vi "11 - Design Pattern - When Generation Rate exceeds Handling Rate (Accumulator).vi"() -> ()   [LabVIEW 2012]
uses:
  <vilib>/Utility/miscctls.llb/LVPoint32TypeDef.ctl
  <vilib>/Utility/miscctls.llb/LVPointTypeDef.ctl
  <vilib>/event_ctls.llb/lveventtype.ctl
panel:
  out "Canvas":picture
  in  "Erase":bool
  out "Events Handled per Update":dbl format="%.02f"
  in  "Handler Throttle Period":u32(ring)=50 items=["None"=0, "50msec"=50, "200msec"=200, "500msec"=500]
  out "Processor Usage":sgl(graph)
  out "Initial Coords":T1
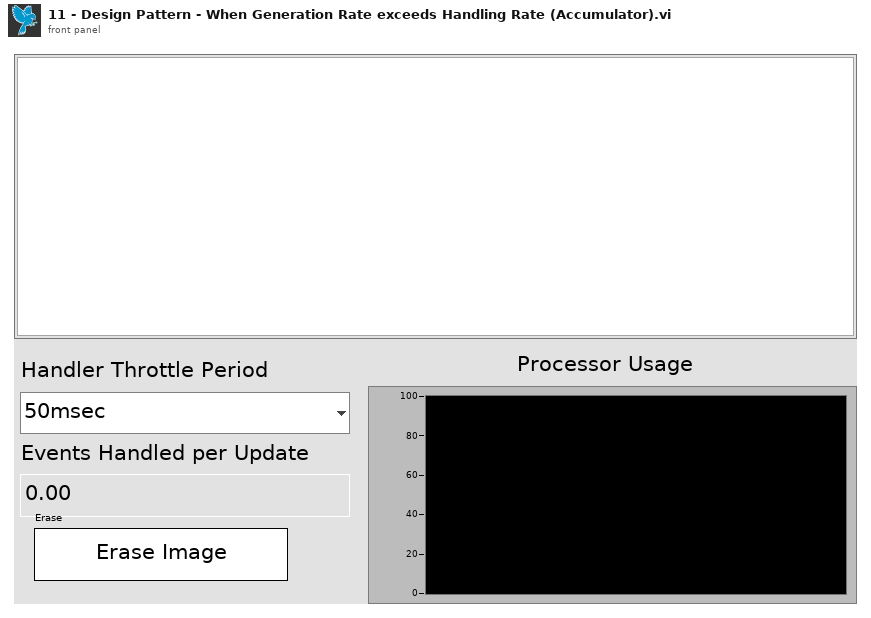
[diagram p1: front panel]
types:
  T1 = typedef "LVPoint32TypeDef.ctl" = cluster{"Horizontal":i32, "Vertical":i32}
  T2 = typedef "LVPointTypeDef.ctl" = cluster{"Horizontal":i16, "Vertical":i16}
  T3 = enum16{"Currently Painting", "Currently Zooming", "No Action"}
  T4 = typedef "lveventtype.ctl" = enum32{"Null", "Timeout", "Annotation Menu Selection", "Annotation Menu Selection?", "App Instance Close", "App Instance Close?", "Autoscale Range Change", "Cell Edit", "Cell Edit?", "Cursor Grab", "Cursor Grab?", "Cursor Menu Selection", "Cursor Menu Selection?", "Cursor Move", "Cursor Release", "Data Change", "Direction Change", "Display State Change", "Drag Ended", "Drag Enter", "Drag Leave", "Drag Over", "Drag Source Update", "Drag Starting", "Drag Starting?", "Drop", "Exec State Change", "Key Down", "Key Down?", "Key Repeat", "Key Repeat?", "Key Up", "Listbox Double Click", "Menu Activation?", "Menu Selection (App)", "Menu Selection? (App)", "Menu Selection (User)", "Mouse Down", "Mouse Down?", "Mouse Enter", "Mouse Leave", "Mouse Move", "Mouse Up", "NI Security User Change (App)", "Pane Size", "Panel Close", "Panel Close?", "Panel Resize", "Plot Attribute Change", "Scale Range Change", "Shortcut Menu Activation?", "Shortcut Menu Selection (App)", "Shortcut Menu Selection? (App)", "Shortcut Menu Selection (User)", "Tree Double Click", "Tree Drag", "Tree Drag?", "Tree Drop", "Tree Drop?", "Tree Item Close", "Tree Item Close?", "Tree Item Open", "Tree Item Open?", "Value Change"}
  T5 = cluster{"Width":u16, "Style":enum32{"Solid", "Dash", "Dot", "DashDot", "DashDotDot"}}
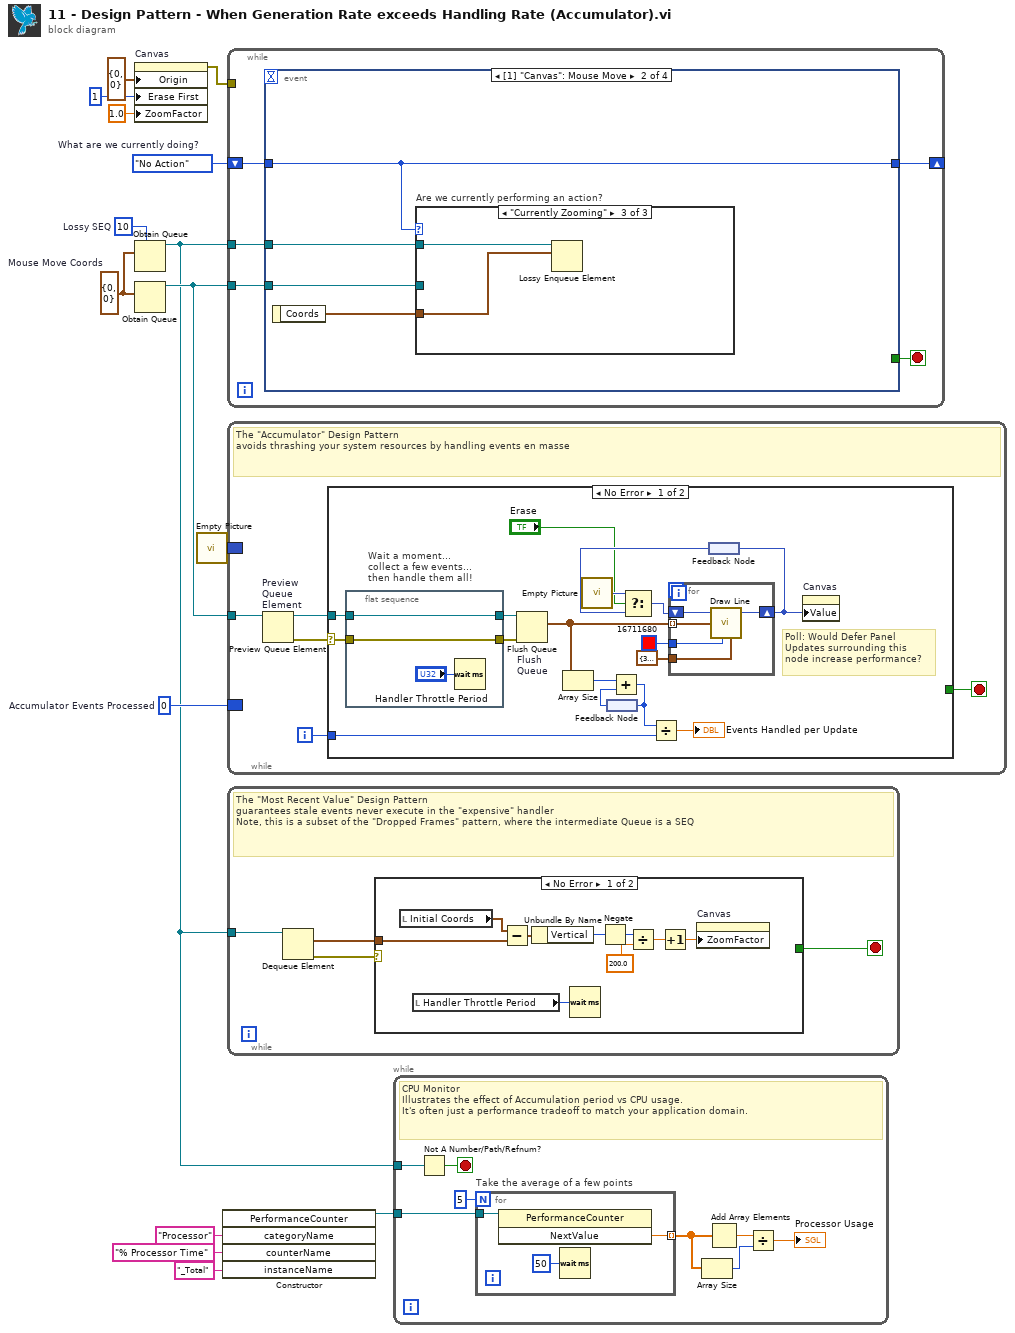
[diagram p0: block diagram]
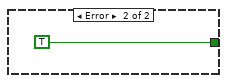
[diagram p2: hidden frame]
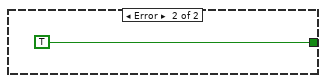
[diagram p3: hidden frame]
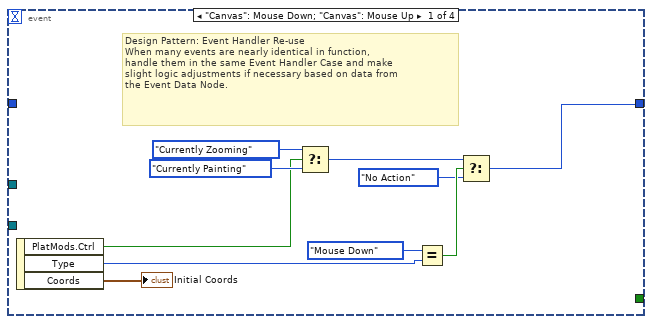
[diagram p4: hidden frame]
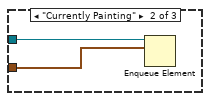
[diagram p6: hidden frame]
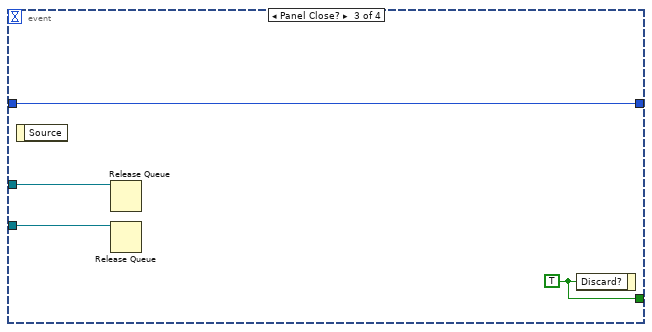
[diagram p7: hidden frame]
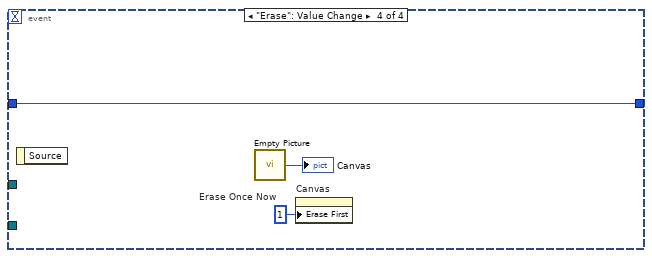
[diagram p8: hidden frame]
diagram:
  w6 = 0  # Accumulator Events Processed
  w14 = 10  # Lossy SEQ
  w15 = T3."No Action"  # What are we currently doing?
  w13 = T1 {"Horizontal"=0, "Vertical"=0}  # Mouse Move Coords
  n1 = property on="Canvas" class="Pict"("Origin"=T2 {"Horizontal"=0, "Vertical"=0}, "Erase First"=u8 1, "ZoomFactor"=sgl 1.0 ("Zoom Factor")) -> (error out=w11:errorcluster)  [unwired: 2 in, 1 out]
  n2 = Obtain Queue(max queue size (-1, unlimited)=w14, element data type=w13) -> (queue out=w2:refnum<queue>)  [unwired: 3 in, 2 out]
  n3 = Obtain Queue(element data type=w13) -> (queue out=w9:refnum<queue>)  [unwired: 4 in, 2 out]
  n4 = call "Empty Picture"() -> ("empty picture"=w10:picture)
  n5 = constructor class="PerformanceCounter"("categoryName"="Processor", "counterName"="% Processor Time", "instanceName"="_Total") -> (reference out=w3:refnum<k24>)  [unwired: 3 in, 5 out]
  n6 = while {
    shift-right: [w19] -> _
    shift-left: w15 -> [w20]
    tunnel: w9 -> [w17]
    tunnel: w2 -> [w16]
    tunnel: w11 -> [_]
    stop <- w18 stop-if-true
    n7 = event shown="[1] \"Canvas\": Mouse Move" {
      selector: _ -> [_ _ _ _]
      dyn-events: _ -> [_ _ _ _]
      timeout: _ -> [_ _ _ _]
      tunnel: w20 -> [_ w32 w41 w45]
      tunnel: [w27 w32 w41 w45] -> w19
      tunnel: [_ _ w42 _] -> w18
      tunnel: w17 -> [_ w34 w39 _]
      tunnel: w16 -> [_ w31 w40 _]
      event "Canvas": Mouse Down; "Canvas": Mouse Up {
        # "Design Pattern: Event Handler Re-use\nWhen many events are nearly identical in function,\nhandle them in the same Event Handler Case and make\nslight logic adjustments if necessary based on data from\nthe Event Data Node."
        n8 = event-data() -> ("PlatMods.Ctrl"=w21:bool, "Type"=w29:T4, "Coords"=→"Initial Coords":T1)  [unwired: 1 in]
        n9 = Select(t=T3."Currently Zooming", s=w21, f=T3."Currently Painting") -> (s? t:f=w25:T3)
        n10 = Equal?(x=lveventtype."Mouse Down" ("Type"), y=w29) -> (x = y?=w28:bool)
        n11 = Select(t=w25, s=w28, f=T3."No Action") -> (s? t:f=w27:T3)
      }
      event "Canvas": Mouse Move {
        n12 = event-data() -> ("Coords"=w33:T1)  [unwired: 1 in]
        n13 = case "Are we currently performing an action?" shown="\"Currently Zooming\"" w32 {
          tunnel: w34 -> [_ w36 _]
          tunnel: w33 -> [_ w35 w38]
          tunnel: w31 -> [_ _ w37]
          frame Default {
          }
          frame "Currently Painting" {
            n14 = Enqueue Element(queue=w36, element=w35) -> ()  [unwired: 2 in, 3 out]
          }
          frame "Currently Zooming" {
            n15 = Lossy Enqueue Element(queue=w37, element=w38) -> ()  [unwired: 1 in, 4 out]
          }
        }
      }
      event Panel Close? {
        w42 = TRUE ("Discard?")
        n16 = event-data() -> ()  [unwired: 1 in, 1 out]
        n17 = Release Queue(queue=w40) -> ()  [unwired: 2 in, 3 out]
        n18 = Release Queue(queue=w39) -> ()  [unwired: 2 in, 3 out]
        n19 = event-data("Discard?"=w42) -> ()  [unwired: 1 in, 1 out]
      }
      event "Erase": Value Change {
        w43 = u8 1  # Erase Once Now
        n20 = event-data() -> ()  [unwired: 1 in, 1 out]
        n21 = call "Empty Picture"() -> ("empty picture"=→"Canvas":picture)
        n22 = property on="Canvas" class="Pict"("Erase First"=w43) -> ()  [unwired: 2 in, 2 out]
      }
    }
  }
  n23 = while {
    tunnel: w9 -> [w50]
    border: w10 -> [_]
    border: w6 -> [_]
    i -> [w46]
    stop <- w47 stop-if-true
    # "The \"Accumulator\" Design Pattern\navoids thrashing your system resources by handling events en masse"
    n24 = Preview Queue Element "Preview\nQueue\nElement"(queue=w50) -> (queue out=w48:refnum<queue>, error out=w49:errorcluster)  [unwired: 2 in, 2 out]
    n25 = case shown="No Error" w49 {
      selector: w49 -> [w66 _]
      tunnel: w48 -> [w65 _]
      tunnel: [_ TRUE] -> w47
      tunnel: w46 -> [w56 _]
      frame No Error {
        # "Poll: Would Defer Panel\nUpdates surrounding this\nnode increase performance?"
        n26 = flat-sequence "Wait a moment...\ncollect a few events...\nthen handle them all!" {
          tunnel: [w75] -> w67
          tunnel: w66 -> [w75]
          tunnel: w65 -> [w74]
          tunnel: [w74] -> w64
          frame #0 {
            n27 = Wait (ms)(milliseconds to wait="Handler Throttle Period") -> ()  [unwired: 1 out]
          }
        }
        n28 = Flush Queue "Flush\nQueue"(queue=w64, error in (no error)=w67) -> (remaining elements=w62:T1[])  [unwired: 2 out]
        n29 = Array Size(array=w62) -> (size(s)=w61:i32)
        n30 = call "Empty Picture"() -> ("empty picture"=w54:picture)
        n31 = feedback #1() -> (w60:i32)
        n32 = Add(x=w61, y=w60) -> (x+y=w57:i32)
        n33 = feedback-in #1(w57) -> ()
        n34 = Divide(x=w57, y=w56) -> (x/y=→"Events Handled per Update":dbl)
        n35 = feedback #2() -> (w53:picture)
        n36 = Select(t=w54, s="Erase", f=w53) -> (s? t:f=w52:picture)
        n37 = for {
          shift-right: [w72] -> w63
          shift-left: w52 -> [w71]
          tunnel: w62 -> [w70] mode=indexing
          tunnel: u32 16711680 ("color(black)") -> [w69]
          tunnel: T5 {"Width"=3, "Style"=enum."Solid"} ("pen") -> [w68]
          n38 = call <vilib>:"Draw Line.vi"("picture"=w71, "end point"=w70, "color(black)"=w69, "pen"=w68) -> ("new picture"=w72:picture)  [unwired: 5 in]
        }
        n39 = feedback-in #2(w63) -> ()
        n40 = property on="Canvas" class="Pict"("Value"=w63) -> ()  [unwired: 2 in, 2 out]
      }
      frame Error {
      }
    }
  }
  n41 = while {
    tunnel: w2 -> [w80]
    stop <- w77 stop-if-true
    # "The \"Most Recent Value\" Design Pattern\nguarantees stale events never execute in the \"expensive\" handler\nNote, this is a subset of the \"Dropped Frames\" pattern, where the intermediate Queue is a SEQ"
    n42 = Dequeue Element(queue=w80) -> (element=w78:T1, error out=w79:errorcluster)  [unwired: 2 in, 2 out]
    n43 = case shown="No Error" w79 {
      tunnel: w78 -> [w89 _]
      tunnel: [_ TRUE] -> w77
      frame No Error {
        n44 = local read "Initial Coords"() -> (w82:T1)
        n45 = local read "Handler Throttle Period"() -> (w86:u32)
        n46 = Subtract(x=w82, y=w89) -> (x-y=w88:T1)
        n47 = Unbundle By Name(w88) -> ("Vertical"=w83:i32)
        n48 = Wait (ms)(milliseconds to wait=w86) -> ()  [unwired: 1 out]
        n49 = Negate(x=w83) -> (-x=w81:i32)
        n50 = Divide(x=w81, y=200.0) -> (x/y=w87:dbl)
        n51 = Increment(x=w87) -> (x+1=w84:dbl)
        n52 = property on="Canvas" class="Pict"("ZoomFactor"=w84) -> ()  [unwired: 2 in, 2 out]
      }
      frame Error {
      }
    }
  }
  n53 = while {
    tunnel: w3 -> [w98]
    tunnel: w2 -> [w97]
    stop <- w96 stop-if-true
    # "CPU Monitor\nIllustrates the effect of Accumulation period vs CPU usage.\nIt's often just a performance tradeoff to match your application domain."
    n54 = Not A Number/Path/Refnum?(number/path/refnum=w97) -> (NaN/Path/Refnum?=w96:bool)
    n55 = for "Take the average of a few points" {
      N: 5 -> [_]
      tunnel: w98 -> [w101]
      tunnel: [w100] -> w94 mode=indexing
      n56 = invoke class="PerformanceCounter" method="NextValue"(reference=w101) -> ("NextValue"=w100:sgl)  [unwired: 2 in, 2 out]
      n57 = Wait (ms)(milliseconds to wait=u32 50) -> ()  [unwired: 1 out]
    }
    n58 = Array Size(array=w94) -> (size(s)=w92:i32)
    n59 = Add Array Elements(numeric array=w94) -> (sum=w93:sgl)
    n60 = Divide(x=w93, y=w92) -> (x/y=→"Processor Usage":sgl)
  }
